vi "Arrays.vi"() -> ()   [LabVIEW 2020]
panel:
  out "Array 2":u8[](array[slide]) scale=0.0..100.0
  in  "Array":dbl[](array[numeric])
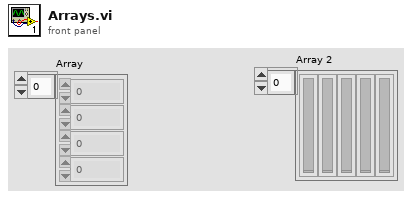
[diagram p1: front panel]
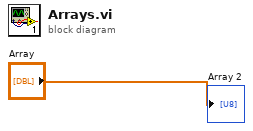
[diagram p0: block diagram]
diagram:
  "Array 2" <- "Array"
